vi "Sine function fitting.vi"(6 "Additional\nLM fitting?":bool=TRUE, 7 "frequency guess":dbl, 8 "error in (no error)":errorcluster caption="Error in", 9 "dt":dbl=1.0, 10 "Input X (null)":dbl[](array[numeric]), 11 "Input Y":dbl[](array[numeric])) -> (0 "error out":errorcluster caption="Error out", 1 "Residue":dbl[](array[numeric]), 2 "best fit parameters":dbl[](array[numeric]) caption="Best Fitt Params", 3 "best nonlinear fit":dbl[](array[numeric]))   [LabVIEW 2020, in "Measure angular gains.lvlib"]
uses:
  Measure angular gains.lvlib
  <vilib>/measure/matone.llb/Extract Single Tone Information 1 Chan.vi
  <vilib>/gmath/NumericalOptimization/Nonlinear Curve Fit LM formula string.vi
  <vilib>/measure/NI_MAPro.lvlib
  <vilib>/gmath/NI_Gmath.lvlib
panel:
  out "y0":dbl
  in  "termination":cluster{"max iteration":i32, "tolerance":dbl}={"max iteration"=200, "tolerance"=1e-08}
  out "Data Fitting":cluster{dbl[], "Input Y":dbl[]}[](graph)
  out "detected frequency":dbl format="%_6g"
  out "detected amplitude":dbl format="%_6g"
  out "detected phase":dbl format="%_6g"
  out "Residues":cluster{dbl[], dbl[]}[](graph)
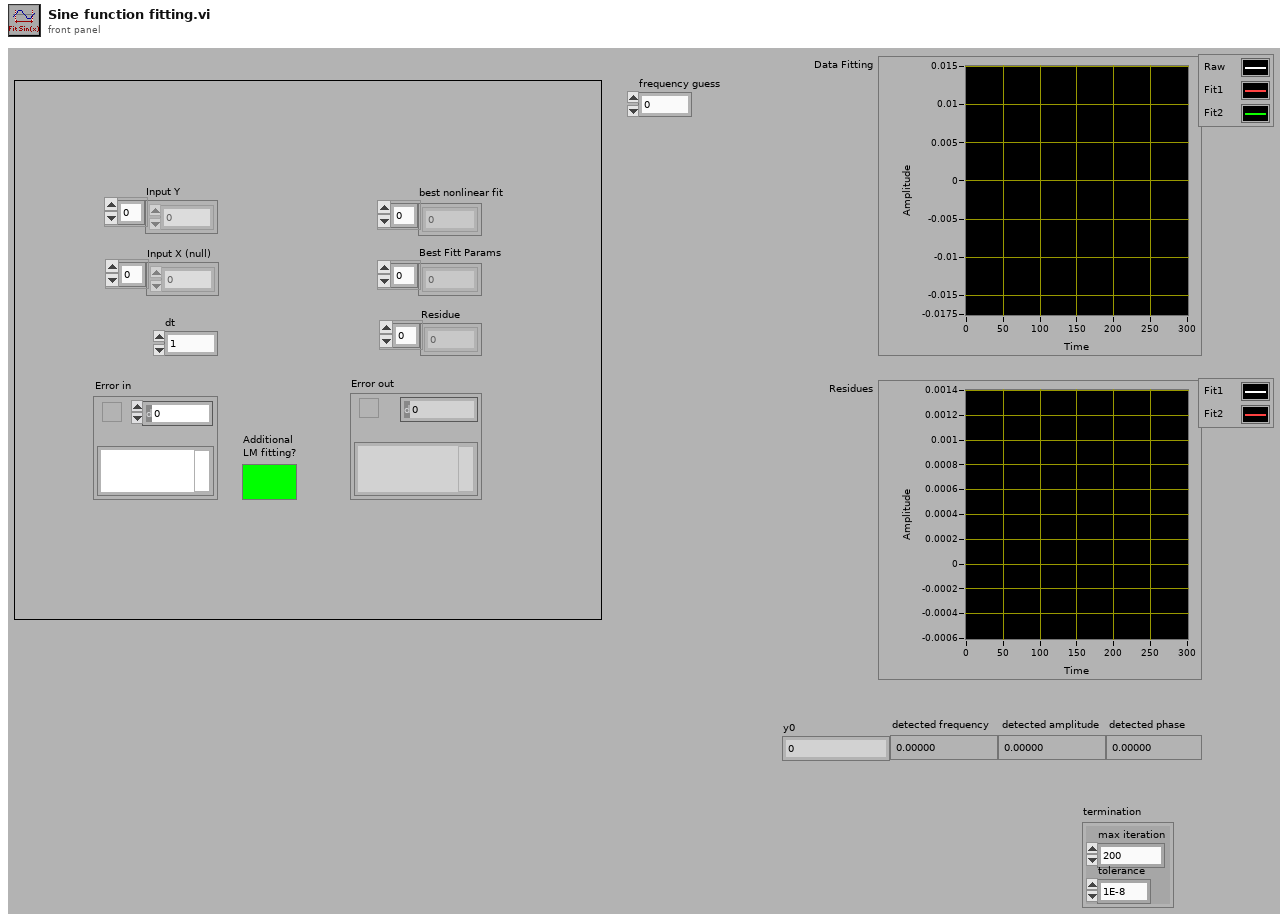
[diagram p1: front panel]
types:
  T1 = cluster{"model":string, "Parameters":string[], "x":string}
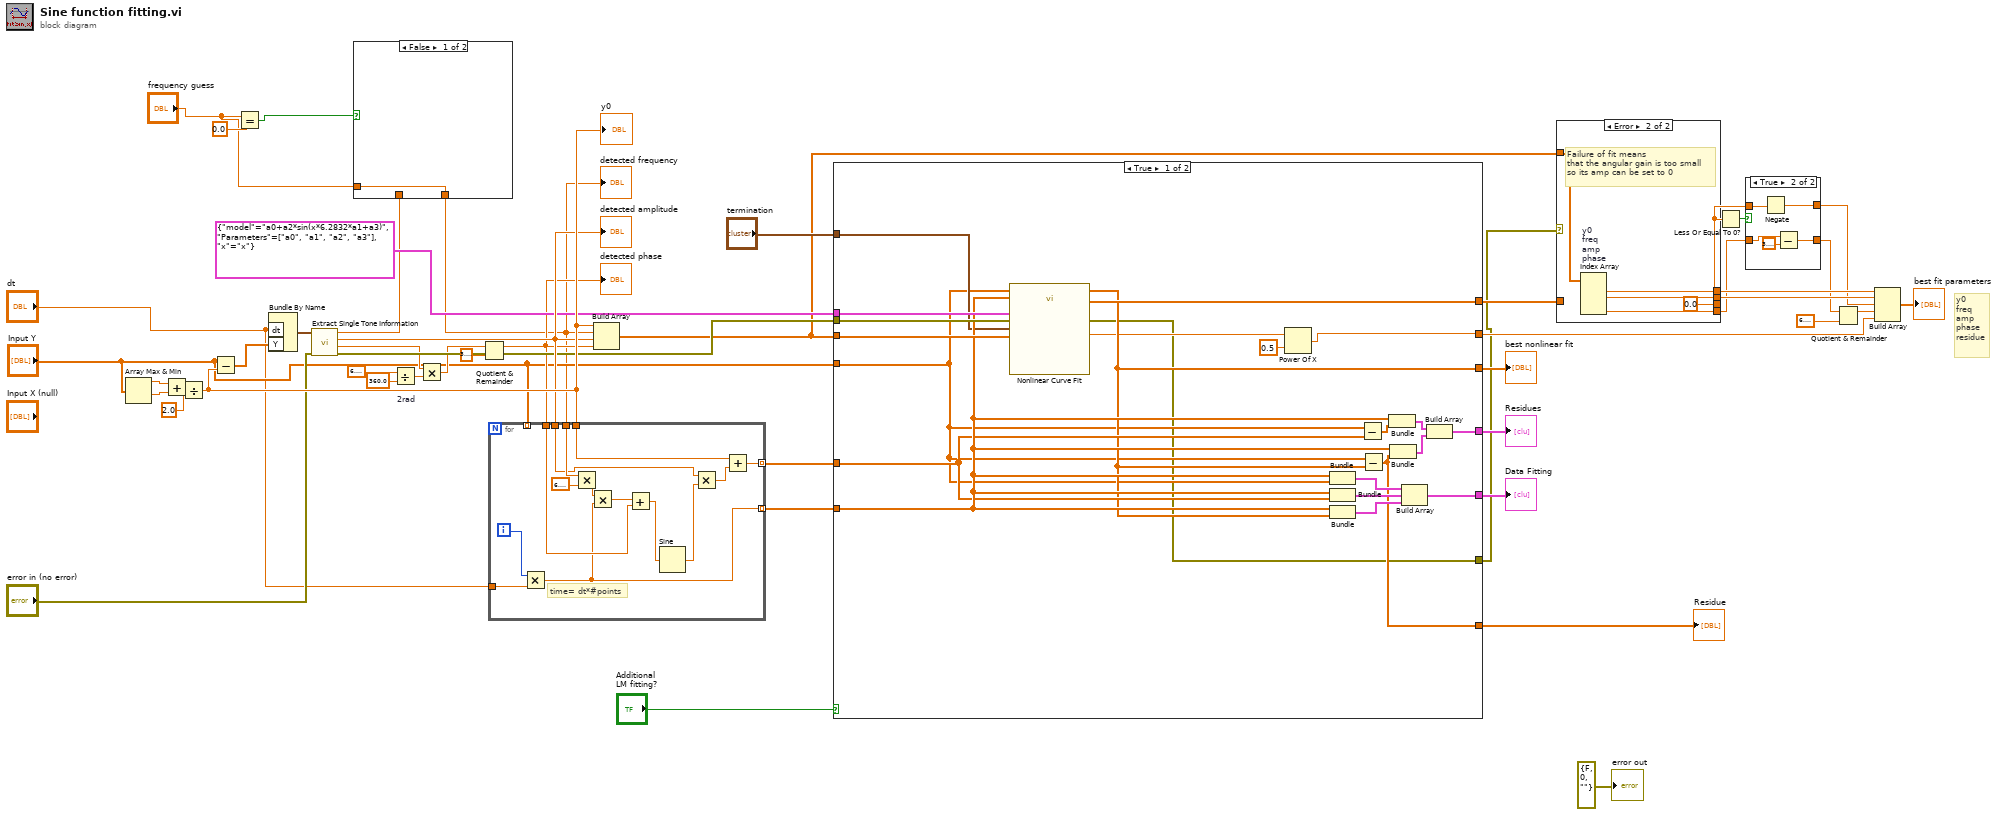
[diagram p0: block diagram]
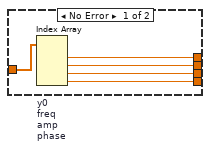
[diagram p3: hidden frame]
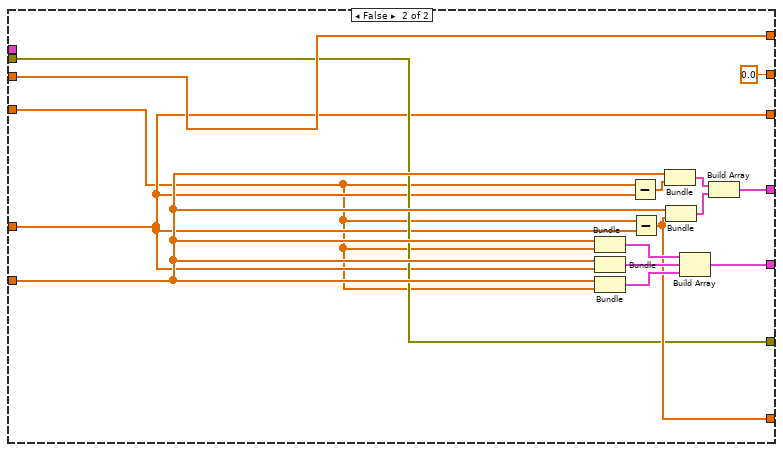
[diagram p5: hidden frame]
diagram:
  # "y0\nfreq\namp\nphase\nresidue"
  n1 = Array Max & Min(array="Input Y") -> (max value=w44:dbl, min value=w45:dbl)  [unwired: 2 out]
  n2 = Add(x=w44, y=w45) -> (x+y=w43:dbl)
  n3 = Divide(x=w43, y=2.0) -> (x/y=w48:dbl)
  "y0" <- w48
  n4 = Subtract(x="Input Y", y=w48) -> (x-y=w41:dbl[])
  n5 = Equal?(x="frequency guess", y=0.0) -> (x = y?=w3:bool)
  n6 = Bundle By Name("dt"="dt", "Y"=w41) -> (w47:waveform(dbl))  [unwired: 1 in]
  n7 = call-poly <vilib>:"Extract Single Tone Information.vi"("error in (no error)"="error in (no error)", "time signal in"=w47) -> ("error out"=w39:errorcluster, "detected phase (deg)"=w28:dbl, "detected amplitude"=w40:dbl, "detected frequency"=w5:dbl)  [unwired: 4 in, 2 out]
  "detected amplitude" <- w40
  n8 = case shown="False" w3 {
    tunnel: w5 -> [_ w50]
    tunnel: [w49 w50] -> w2
    tunnel: "frequency guess" -> [w49 _]
    frame False {
    }
    frame True {
    }
  }
  "detected frequency" <- w2
  n9 = Divide "2rad"(x=6.283185307179586, y=360.0) -> (x/y=w29:dbl)
  n10 = Multiply(x=w28, y=w29) -> (x*y=w25:dbl)
  n11 = Quotient & Remainder(x=w25, y=3.141592653589793) -> (x-y*floor(x/y)=w24:dbl)  [unwired: 1 out]
  "detected phase" <- w24
  n12 = for {
    tunnel: [w51] -> w36 mode=indexing
    tunnel: w2 -> [w64]
    tunnel: w40 -> [w61]
    tunnel: w24 -> [w58]
    tunnel: [w54] -> w35 mode=indexing
    tunnel: "Input Y" -> [_] mode=indexing
    tunnel: w48 -> [w56]
    tunnel: "dt" -> [w53]
    i -> [w52]
    # "time= dt*#points"
    n13 = Multiply(x=w52, y=w53) -> (x*y=w51:dbl)
    n14 = Multiply(x=w64, y=6.283185307179586) -> (x*y=w63:dbl)
    n15 = Multiply(x=w63, y=w51) -> (x*y=w62:dbl)
    n16 = Add(x=w62, y=w58) -> (x+y=w60:dbl)
    n17 = Sine(x=w60) -> (sin(x)=w59:dbl)
    n18 = Multiply(x=w61, y=w59) -> (x*y=w55:dbl)
    n19 = Add(x=w56, y=w55) -> (x+y=w54:dbl)
  }
  n20 = Build Array(w48, w2, w40, w24) -> (w7:dbl[])
  n21 = case shown="True" "Additional\nLM fitting?" {
    tunnel: [w86 w101] -> w46
    tunnel: w7 -> [w85 w91]
    tunnel: w39 -> [w84 w90]
    tunnel: T1 {"model"="a0+a2*sin(x*6.2832*a1+a3)", "Parameters"=["a0", "a1", "a2", "a3"], "x"="x"} ("model description") -> [w83 _]
    tunnel: [w79 w91] -> w23
    tunnel: [w77 w96] -> w18
    tunnel: [w76 w95] -> w37
    tunnel: w36 -> [w75 w94]
    tunnel: w35 -> [w74 w89]
    tunnel: [w73 w89] -> w34
    tunnel: [w65 w90] -> w6
    tunnel: "termination" -> [w70 _]
    tunnel: "Input Y" -> [w69 w88]
    tunnel: [w67 0.0 ("residue")] -> w17
    frame True {
      n22 = call-poly <vilib>:"Nonlinear Curve Fit.vi"("Y"=w69, "initial parameters"=w85, "X"=w75, "model description"=w83, "error in (no error)"=w84, "termination"=w70) -> ("best nonlinear fit"=w73:dbl[], "best fit parameters"=w79:dbl[], "residue"=w68:dbl, "error out"=w65:errorcluster)  [unwired: 5 in, 1 out]
      n23 = Power Of X(1:0.5 ("x"), 2:w68) -> (0:w67:dbl)
      n24 = Bundle(w75, "Input Y"=w69) -> (w81:cluster{dbl[], "Input Y":dbl[]})  [unwired: 1 in]
      n25 = Bundle(w75, w74) -> (w82:cluster{dbl[], dbl[]})  [unwired: 1 in]
      n26 = Bundle(w75, "best nonlinear fit"=w73) -> (w80:cluster{dbl[], "best nonlinear fit":dbl[]})  [unwired: 1 in]
      n27 = Subtract(x=w69, y=w74) -> (x-y=w78:dbl[])
      n28 = Subtract(x=w69, y=w73) -> (x-y=w77:dbl[])
      n29 = Bundle(w75, w78) -> (w72:cluster{dbl[], dbl[]})  [unwired: 1 in]
      n30 = Bundle(w75, w77) -> (w71:cluster{dbl[], dbl[]})  [unwired: 1 in]
      n31 = Build Array(w81, w82, w80) -> (w86:cluster{dbl[], "best nonlinear fit":dbl[]}[])
      n32 = Build Array(w72, w71) -> (w76:cluster{dbl[], dbl[]}[])
    }
    frame False {
      n33 = Bundle(w94, "Input Y"=w88) -> (w99:cluster{dbl[], "Input Y":dbl[]})  [unwired: 1 in]
      n34 = Bundle(w94, w89) -> (w100:cluster{dbl[], dbl[]})  [unwired: 1 in]
      n35 = Bundle(w94, "Input Y"=w88) -> (w98:cluster{dbl[], "Input Y":dbl[]})  [unwired: 1 in]
      n36 = Subtract(x=w88, y=w89) -> (x-y=w97:dbl[])
      n37 = Subtract(x=w88, y=w89) -> (x-y=w96:dbl[])
      n38 = Bundle(w94, w97) -> (w93:cluster{dbl[], dbl[]})  [unwired: 1 in]
      n39 = Bundle(w94, w96) -> (w92:cluster{dbl[], dbl[]})  [unwired: 1 in]
      n40 = Build Array(w99, w100, w98) -> (w101:cluster{dbl[], "Input Y":dbl[]}[])
      n41 = Build Array(w93, w92) -> (w95:cluster{dbl[], dbl[]}[])
    }
  }
  "Data Fitting" <- w46
  "Residues" <- w37
  "best nonlinear fit" <- w34
  "Residue" <- w18
  n42 = case shown="Error" w6 {
    tunnel: w23 -> [w106 _]
    tunnel: [w105 w111] -> w22
    tunnel: [w104 w110] -> w21
    tunnel: [w103 w109] -> w15
    tunnel: [w102 0.0 ("detected amplitude")] -> w14
    tunnel: w7 -> [_ w108]
    frame No Error {
      n43 = Index Array "y0\nfreq\namp\nphase"(array=w106) -> (element #1=w105:dbl, element #2=w104:dbl, element #3=w102:dbl, element #4=w103:dbl)  [unwired: 4 in]
    }
    frame Error {
      # "Failure of fit means\nthat the angular gain is too small\nso its amp can be set to 0"
      n44 = Index Array "y0\nfreq\namp\nphase"(array=w108) -> (element #1=w111:dbl, element #2=w110:dbl, element #4=w109:dbl)  [unwired: 4 in, 1 out]
    }
  }
  n45 = Less Or Equal To 0?(x=w14) -> (x <= 0?=w16:bool)
  n46 = case shown="True" w16 {
    tunnel: w15 -> [w112 w116]
    tunnel: w14 -> [w113 w118]
    tunnel: [w113 w117] -> w13
    tunnel: [w112 w114] -> w12
    frame False {
    }
    frame True {
      n47 = Negate(x=w118) -> (-x=w117:dbl)
      n48 = Subtract(x=w116, y=3.141592653589793) -> (x-y=w114:dbl)
    }
  }
  n49 = Quotient & Remainder(x=w12, y=6.283185307179586) -> (x-y*floor(x/y)=w20:dbl)  [unwired: 1 out]
  n50 = Build Array(w22, w21, w13, w20, w17) -> (→"best fit parameters":dbl[])
  "error out" <- errorcluster {"status"=FALSE, "code"=0, "source"=""} ("error out")
